vi "Get Document.Path.vi"(8 "error in (no error)":errorcluster, 11 "npoiDocument in":refnum<class "npoiDocument.lvclass">) -> (0 "error out":errorcluster, 2 "Document.Path":path, 3 "npoiDocument out":refnum<class "npoiDocument.lvclass">)   [LabVIEW 2017, in "NPOI_Document.lvlib" / "npoiDocument.lvclass"]
uses:
  npoiDocument.lvclass
  npoiDocument.lvclass/npoiDocument.ctl
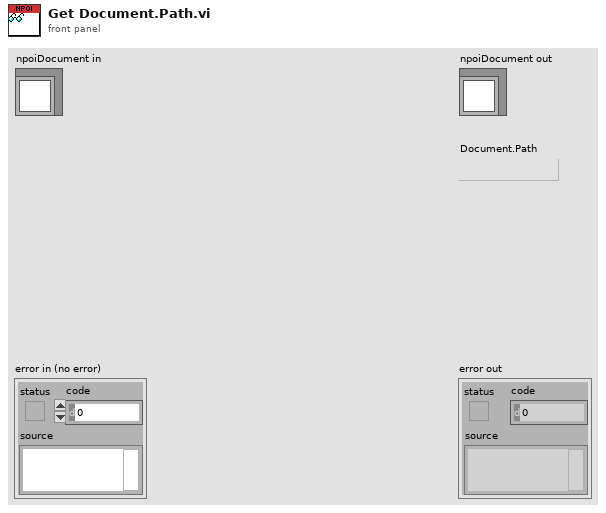
[diagram p1: front panel]
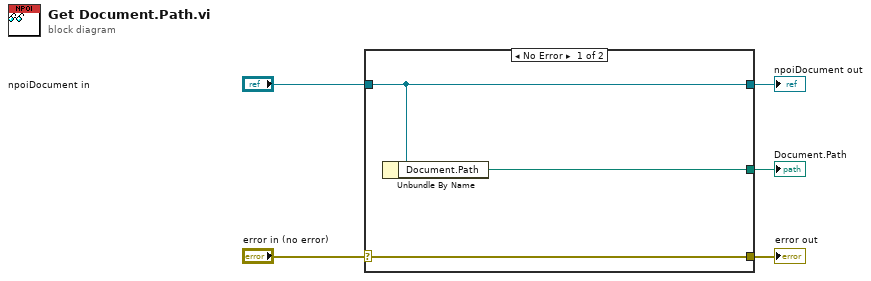
[diagram p0: block diagram]
diagram:
  n1 = case shown="No Error" "error in (no error)" {
    selector: "error in (no error)" -> [w8 w9]
    tunnel: [w8 w9] -> w4
    tunnel: [w7 w10] -> w2
    tunnel: "npoiDocument in" -> [w7 w10]
    tunnel: [w6 _] -> w1
    frame No Error {
      n2 = Unbundle By Name(w7) -> ("Document.Path"=w6:path)
    }
    frame Error {
    }
  }
  "error out" <- w4
  "npoiDocument out" <- w2
  "Document.Path" <- w1
